vi "collimator_GUI.vi"(4 "error in (no error)":errorcluster, 7 "connection ID":refnum<k5>) -> (0 "error out":errorcluster)   [LabVIEW 2015]
doc: "Use this template to build a PDA VI for Pocket PC 2002 devices or emulators."
panel:
  in  "Cancel":bool
  in  "OK":bool
  in  "Focus":i32
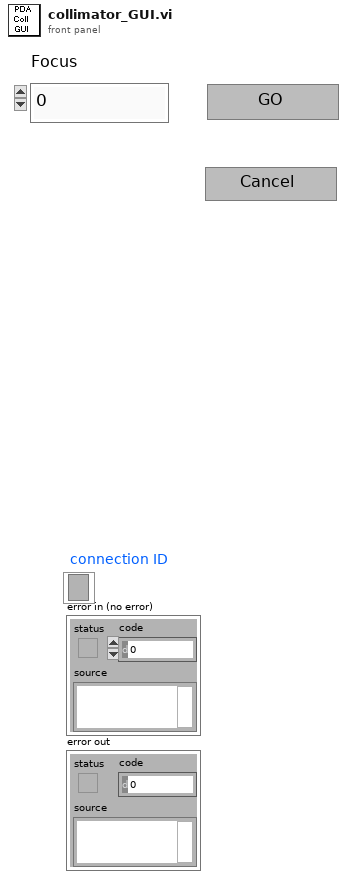
[diagram p1: front panel]
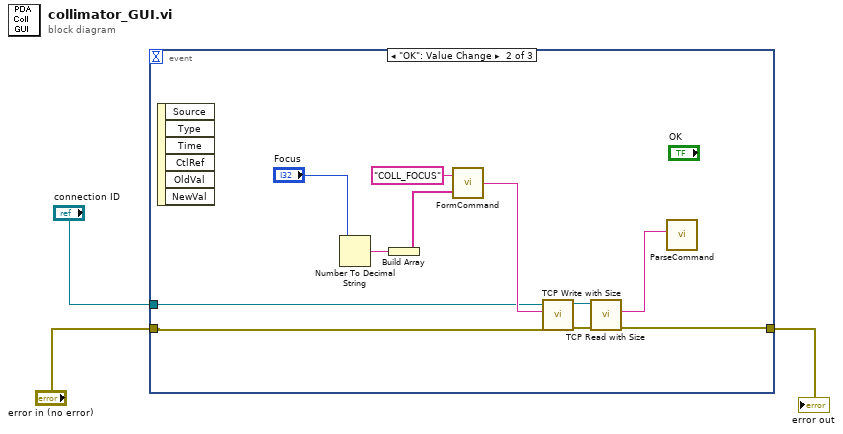
[diagram p0: block diagram]
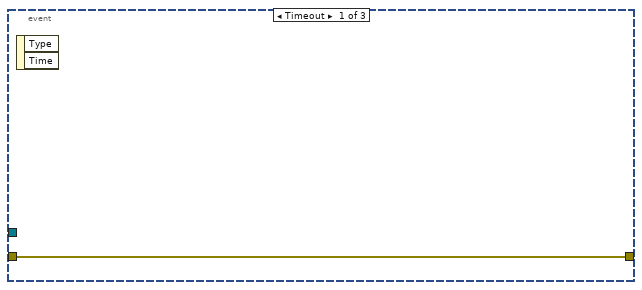
[diagram p2: hidden frame]
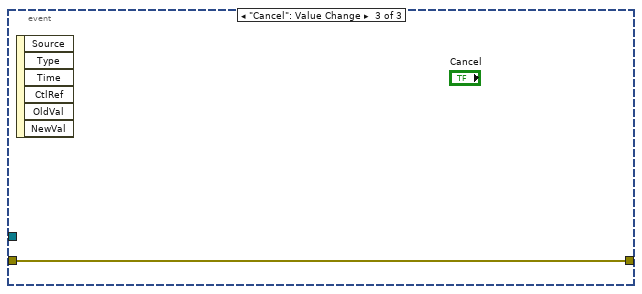
[diagram p3: hidden frame]
diagram:
  n1 = event shown="[1] \"OK\": Value Change" {
    selector: _ -> [_ _ _]
    dyn-events: _ -> [_ _ _]
    timeout: _ -> [_ _ _]
    tunnel: "connection ID" -> [_ w8 _]
    tunnel: "error in (no error)" -> [w4 w7 w16]
    tunnel: [w4 w6 w16] -> w1
    event Timeout {
      n2 = event-data() -> ()  [unwired: 1 in, 2 out]
    }
    event "OK": Value Change {
      n3 = event-data() -> ()  [unwired: 1 in, 6 out]
      n4 = Number To Decimal String(number="Focus") -> (decimal integer string=w14:string)  [unwired: 1 in]
      n5 = Build Array(w14) -> (w13:string[])
      n6 = call "FormCommand.vi"("Parameters"=w13, "Command"="COLL_FOCUS") -> ("Command string"=w12:string)
      n7 = call "TCP Write with Size.vi"("error in (no error)"=w7, "data in"=w12, "connection ID"=w8) -> ("error out"=w11:errorcluster, "connection ID out"=w10:refnum<k5>)  [unwired: 6 in, 1 out]
      n8 = call "TCP Read with Size.vi"("error in (no error)"=w11, "connection ID"=w10) -> ("error out"=w6:errorcluster, "data out"=w9:string)  [unwired: 7 in, 1 out]
      n9 = call "ParseCommand.vi"("Command string"=w9) -> ()  [unwired: 2 out]
    }
    event "Cancel": Value Change {
      n10 = event-data() -> ()  [unwired: 1 in, 6 out]
    }
  }
  "error out" <- w1
